vi "LS_372_start_ramping.vi"(6 "Channel":u16, 7 "VISA-Ressourcenname":refnum<visa-resource-name>) -> (3 "Setpoint":dbl)   [LabVIEW 2019]
uses:
  Global/Global Variables/global.vi
  Global/Global Variables/Data_Display_global.vi
  Equipment/Lake Shore 372/Lake Shore 372.lvlib
panel:
  in  "Warmup % (50%)":dbl=50.0 min=0.0 max=100.0 step=1.0
  in  "Setpoint Change Delay (25sec)":i32=25 min=1 max=255 step=1
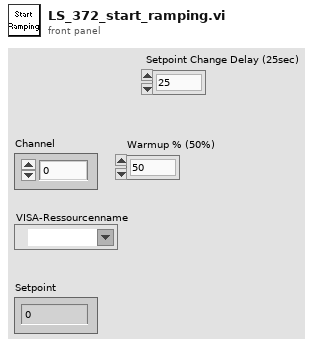
[diagram p1: front panel]
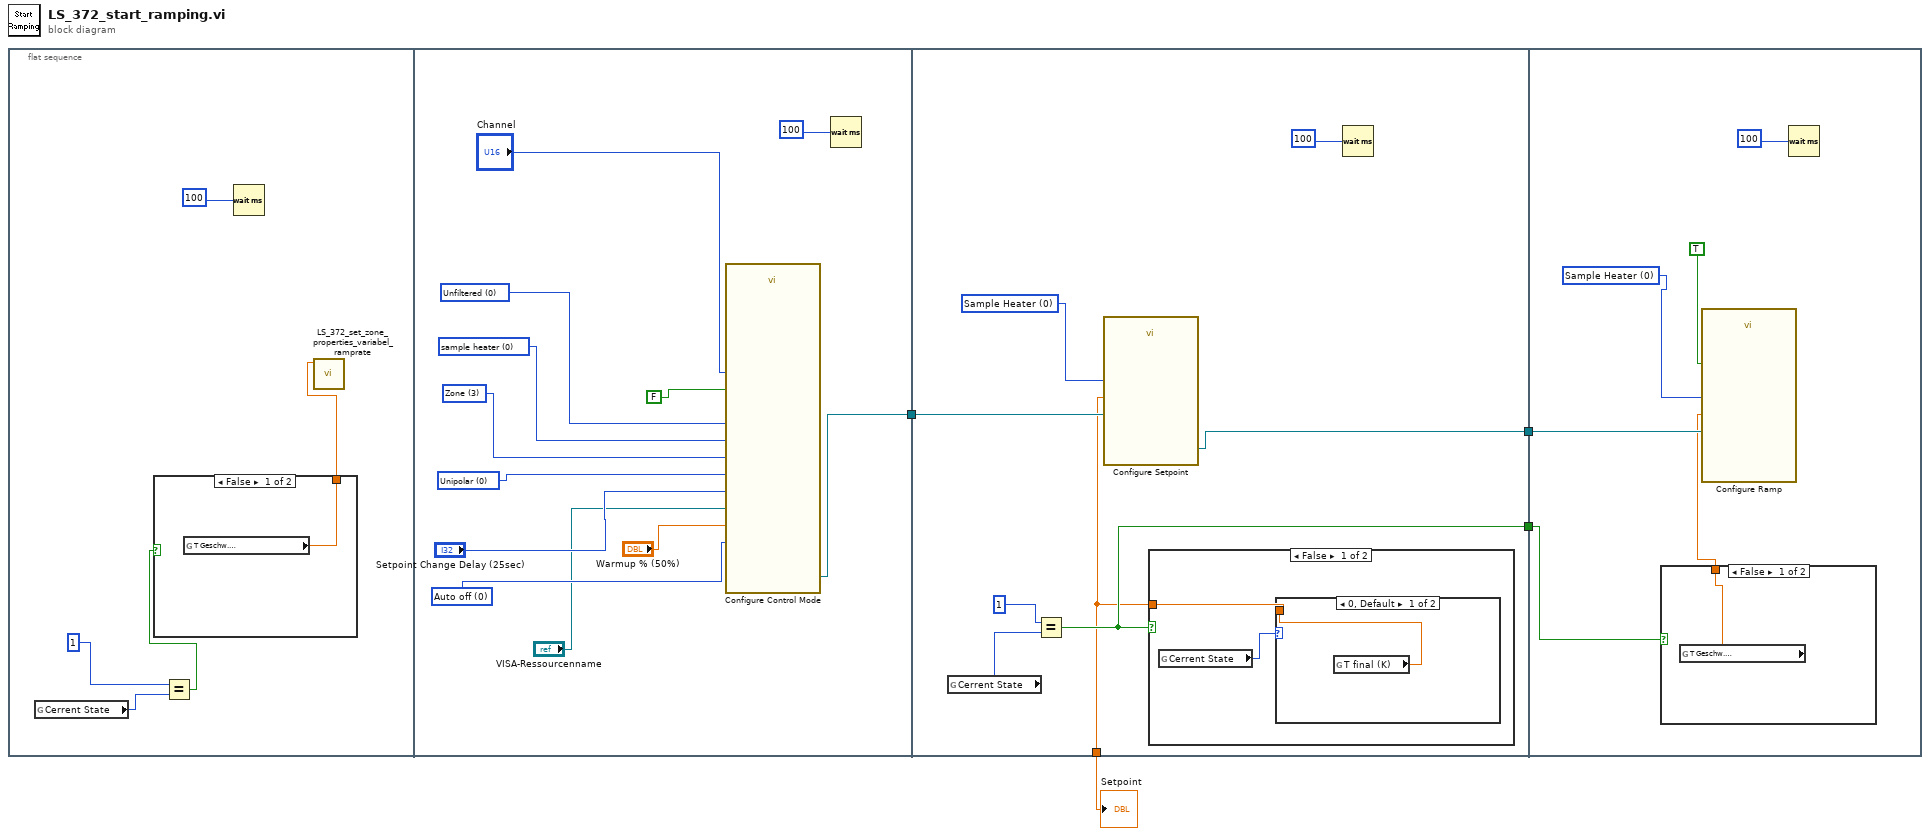
[diagram p0: block diagram]
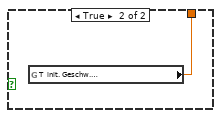
[diagram p2: hidden frame]
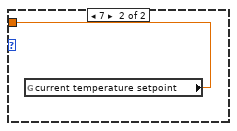
[diagram p3: hidden frame]
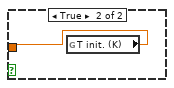
[diagram p4: hidden frame]
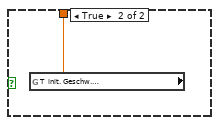
[diagram p5: hidden frame]
diagram:
  n1 = flat-sequence {
    tunnel: [w14] -> w4
    tunnel: w4 -> [w31]
    tunnel: [w28] -> w3
    tunnel: [w27] -> w2
    tunnel: [w26] -> w1
    tunnel: w3 -> [w40]
    tunnel: w1 -> [w41]
    frame #0 {
      n2 = global read "global.vi" "Cerrent State"() -> (w8:i32)
      n3 = Equal?(x=1, y=w8) -> (x = y?=w6:bool)
      n4 = case shown="False" w6 {
        tunnel: [w10 w11] -> w9
        frame False {
          n5 = global read "global.vi" "T Geschw. \n(K/min)"() -> (w10:dbl)
        }
        frame True {
          n6 = global read "global.vi" "T  init. Geschw. \n(K/min)"() -> (w11:dbl)
        }
      }
      n7 = Wait (ms)(milliseconds to wait=100) -> ()  [unwired: 1 out]
      n8 = call "LS_372_set_zone_properties_variabel_ramprate.vi"("Ramprate"=w9) -> ()  [unwired: 11 in]
    }
    frame #1 {
      w17 = u16 0 items=["Auto off", "Continuous"] ("Warmup Control (0: Auto off)")
      w19 = u16 0 items=["Unfiltered", "Filtered"] ("Filtered Readings (0: Unfiltered)")
      w21 = u16 0 items=["Unipolar", "Bipolar"] ("Polarity (0: Unipolar)")
      w22 = u16 0 items=["sample heater", "output 1 (warm-up heater) ", "output 2 (analog/still)"] ("Output (0: sample heater)")
      w23 = u16 3 items=["Off", "Monitor Out", "Open Loop (Manual)", "Zone", "Still", "Closed Loop (PID)", "Warm-up"] ("Output Mode (0: Off)")
      n9 = call "Configure Control Mode.vi"("VISA resource name"="VISA-Ressourcenname", "Enable Power-up (F: Disable)"=FALSE, "Setpoint Change Delay (25sec)"="Setpoint Change Delay (25sec)", "Output (0: sample heater)"=w22, "Channel (1:1)"="Channel", "Output Mode (0: Off)"=w23, "Polarity (0: Unipolar)"=w21, "Filtered Readings (0: Unfiltered)"=w19, "Warmup Control (0: Auto off)"=w17, "Warmup % (50%)"="Warmup % (50%)") -> ("VISA resource name out"=w14:refnum<visa-resource-name>)  [unwired: 4 in, 1 out]
      n10 = Wait (ms)(milliseconds to wait=100) -> ()  [unwired: 1 out]
    }
    frame #2 {
      w24 = u16 0 items=["Sample Heater ", "Warm-up Heater "] ("Output (0: Sample Heater)")
      n11 = global read "global.vi" "Cerrent State"() -> (w29:i32)
      n12 = Equal?(x=1, y=w29) -> (x = y?=w28:bool)
      n13 = case shown="False" w28 {
        tunnel: [w32 w36] -> w27
        frame False {
          n14 = global read "global.vi" "Cerrent State"() -> (w33:i32)
          n15 = case shown="0, Default" w33 {
            tunnel: [w34 w35] -> w32
            frame 0, Default {
              n16 = global read "global.vi" "T final (K)"() -> (w34:dbl)
            }
            frame 7 {
              n17 = global read "Data_Display_global.vi" "current temperature setpoint"() -> (w35:dbl)
            }
          }
        }
        frame True {
          n18 = global read "global.vi" "T init. (K)"() -> (w36:dbl)
        }
      }
      n19 = call "Configure Setpoint.vi"("Setpoint (0.00000E+0)"=w27, "Output (0: Sample Heater)"=w24, "VISA resource name"=w31) -> ("VISA resource name out"=w26:refnum<visa-resource-name>)  [unwired: 7 in, 1 out]
      n20 = Wait (ms)(milliseconds to wait=100) -> ()  [unwired: 1 out]
    }
    frame #3 {
      w42 = u16 0 items=["Sample Heater ", "Warm-up Heater "] ("Output (0: Sample Heater)")
      n21 = case shown="False" w40 {
        tunnel: [w43 w44] -> w39
        frame False {
          n22 = global read "global.vi" "T Geschw. \n(K/min)"() -> (w43:dbl)
        }
        frame True {
          n23 = global read "global.vi" "T  init. Geschw. \n(K/min)"() -> (w44:dbl)
        }
      }
      n24 = call "Configure Ramp.vi"("Rate Value (0.001)"=w39, "Enable Ramping (F: Disable)"=TRUE, "Output (0: Sample Heater)"=w42, "VISA resource name"=w41) -> ()  [unwired: 6 in, 2 out]
      n25 = Wait (ms)(milliseconds to wait=100) -> ()  [unwired: 1 out]
    }
  }
  "Setpoint" <- w2
